vi "Session_Parser.vi"(8 "Error In":errorcluster, 11 "Consumer Data In":T2={"Queue_Consumer"=refnum, "Selected Consumer"=enum."Random", "Session Data"={"Tx-Data"=[], "Rx-Data"=[], "MIDI-Message log"=[{"Message Name"="", "Meta value"=0, "Datastring"="", "Datatype"=enum."No Data"}]}, "Timout-Time[ms]"=0, "To_GUI-Consumer"=refnum, "CPU(ms)"=0, "Console log"="", "MIDI Parse Data"={"MIDI-Bytes In"=[145, 60, 100], "MIDI Tag"=[], "MIDI Parsed Data"=[], "Iteration"=0, "Error?"=[], "Running States"=[], "Running Statusbyte"=0, "Running StatusString"="", "Third Byte Flag"=FALSE, "Current Byte"=0, "Sysex"="", "Expect Databyte"=FALSE}, "Session Inspection Data"={"Diff"=[], "Tx Byte"=[], "Rx Byte"=[], "Send Log"=[], "Parsed Data"={"Tx MIDI Tag"=[], "Tx MIDI Parsed Data"=[], "Tx Error"=[], "Tx Running States"=[], "Rx MIDI Tag"=[], "Rx MIDI Parsed Data"=[], "Rx Error"=[], "Rx Running States"=[], "Diff"=[]}}} {"MIDI Parse Data"."Current Byte" format="%.0x"; "MIDI Parse Data"."Running Statusbyte" format="%.0x"; "MIDI Parse Data"."MIDI-Bytes In" format="%.0x"}) -> (0 "Error Out":errorcluster, 3 "Consumer Data Out":T2={"Queue_Consumer"=refnum, "Selected Consumer"=enum."Random", "Session Data"={"Tx-Data"=[], "Rx-Data"=[], "MIDI-Message log"=[{"Message Name"="", "Meta value"=0, "Datastring"="", "Datatype"=enum."No Data"}]}, "Timout-Time[ms]"=0, "To_GUI-Consumer"=refnum, "CPU(ms)"=0, "Console log"="", "MIDI Parse Data"={"MIDI-Bytes In"=[145, 60, 100], "MIDI Tag"=[], "MIDI Parsed Data"=[], "Iteration"=0, "Error?"=[], "Running States"=[], "Running Statusbyte"=0, "Running StatusString"="", "Third Byte Flag"=FALSE, "Current Byte"=0, "Sysex"="", "Expect Databyte"=FALSE}, "Session Inspection Data"={"Diff"=[], "Tx Byte"=[], "Rx Byte"=[], "Send Log"=[], "Parsed Data"={"Tx MIDI Tag"=[], "Tx MIDI Parsed Data"=[], "Tx Error"=[], "Tx Running States"=[], "Rx MIDI Tag"=[], "Rx MIDI Parsed Data"=[], "Rx Error"=[], "Rx Running States"=[], "Diff"=[]}}} {"MIDI Parse Data"."Current Byte" format="%.0x"; "MIDI Parse Data"."Running Statusbyte" format="%.0x"; "MIDI Parse Data"."MIDI-Bytes In" format="%.0x"})   [LabVIEW 2019]
doc: "Description of VI"
uses:
  Controls/Consumer_Data.ctl
  Common/Controls/Application_Message.ctl
  Common/Controls/Application_State.ctl
  Controls/Consumer_States.ctl
  Controls/Transfer_Data.ctl
  MIDI/Controls/MIDI-Message_Array.ctl
  MIDI/Controls/MIDI-Message_Cluster.ctl
  MIDI/Controls/Meta_Commands.ctl
  Controls/Parser-data.ctl
  Controls/Consumer_Result.ctl
  Controls/Parsed_Data.ctl
  <vilib>/Utility/error.llb/DialogType.ctl
panel:
  out "Control Tab":T1(tab)
  out "Error Message":string
  out "VI-filename":string
  out "VI Path":path
  out "Code Size":u32
  out "Revision Number":u32
  in  "Tool Bar:Visible":bool
  in  "Tabs Visible?":bool
  out "VI-Name":string
  # "Settings"
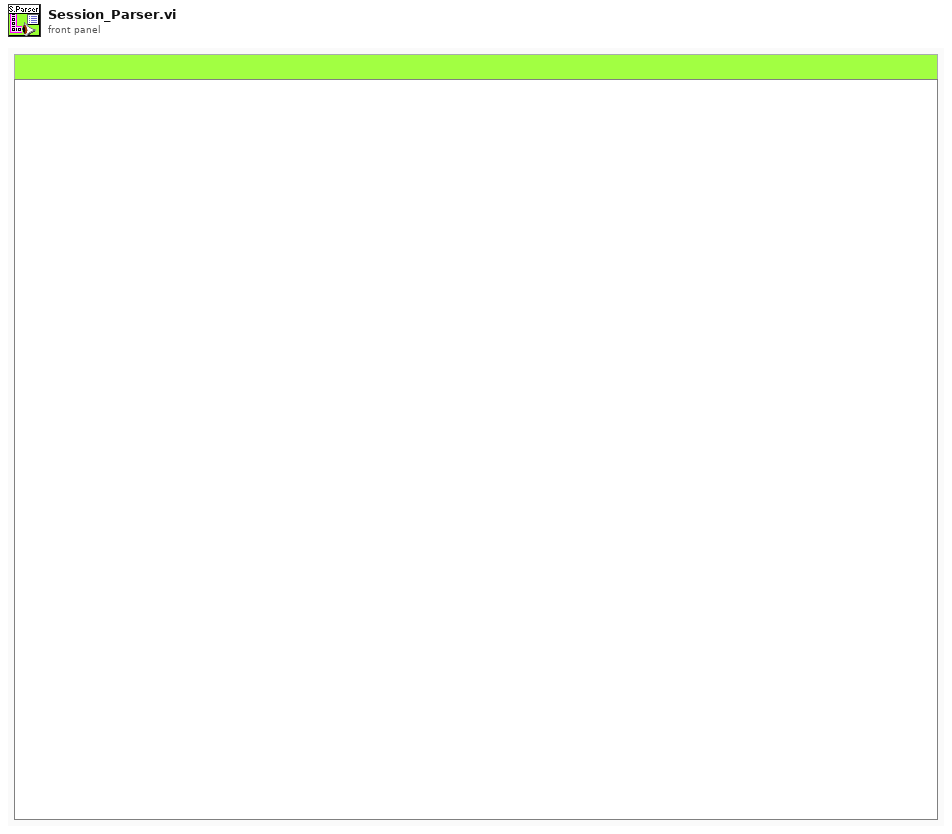
[diagram p1: front panel]
types:
  T1 = enum32{"GUI", "Console Log", "Controls & Indicators", "Data In", "Data Out", "Error IO", "VI"}
  T2 = typedef "Consumer_Data.ctl" = cluster{"Queue_Consumer":refnum<queue>, "Selected Consumer":T3, "Session Data":T4, "Timout-Time[ms]":i32, "To_GUI-Consumer":refnum<user-event>, "CPU(ms)":u32, "Console log":string, "MIDI Parse Data":T8, "Session Inspection Data":T9}
  T3 = typedef "Consumer_States.ctl" = enum16{"Random", "ECG", "Strech-Patch"}
  T4 = typedef "Transfer_Data.ctl" = cluster{"Tx-Data":i8[], "Rx-Data":i8[], "MIDI-Message log":T5}
  T5 = typedef "MIDI-Message_Array.ctl" = T6[]
  T6 = typedef "MIDI-Message_Cluster.ctl" = cluster{"Message Name":string, "Meta value":i32, "Datastring":string, "Datatype":T7}
  T7 = typedef "Meta_Commands.ctl" = enum16{"No Data", "Pause", "Loop", "Wait for Rx", "Delay", "Break", "MIDI"}
  T8 = typedef "Parser-data.ctl" = cluster{"MIDI-Bytes In":u8[], "MIDI Tag":string[], "MIDI Parsed Data":string[], "Iteration":i32, "Error?":bool[], "Running States":string[], "Running Statusbyte":u8, "Running StatusString":string, "Third Byte Flag":bool, "Current Byte":u8, "Sysex":string, "Expect Databyte":bool}
  T9 = typedef "Consumer_Result.ctl" = cluster{"Diff":bool[], "Tx Byte":string[], "Rx Byte":string[], "Send Log":string[], "Parsed Data":T10}
  T10 = typedef "Parsed_Data.ctl" = cluster{"Tx MIDI Tag":string[], "Tx MIDI Parsed Data":string[], "Tx Error":bool[], "Tx Running States":string[], "Rx MIDI Tag":string[], "Rx MIDI Parsed Data":string[], "Rx Error":bool[], "Rx Running States":string[], "Diff":bool[]}
  T11 = typedef "DialogType.ctl" = u16
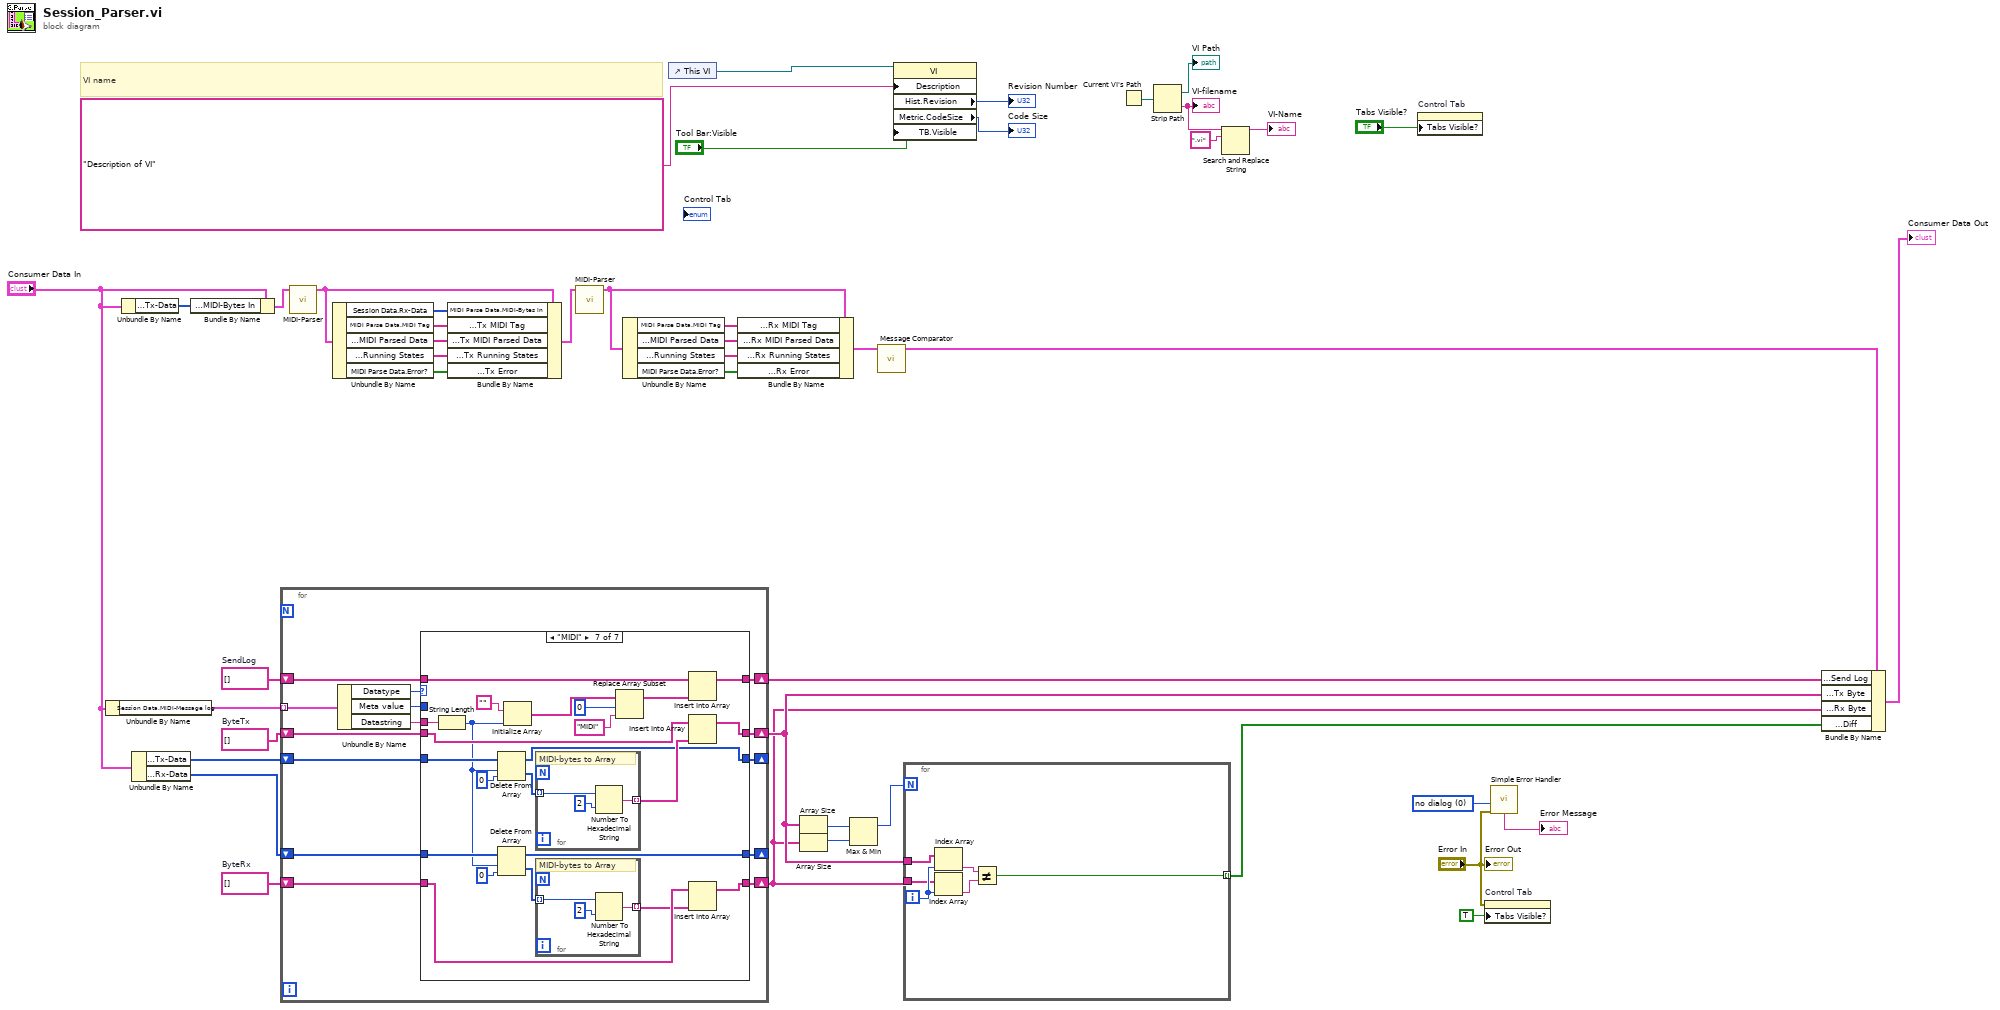
[diagram p0: block diagram]
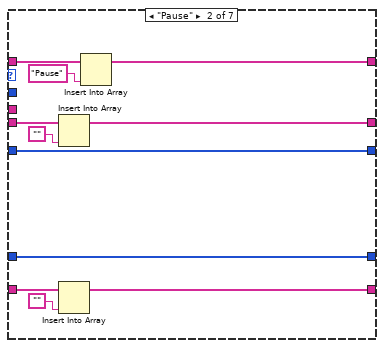
[diagram p3: hidden frame]
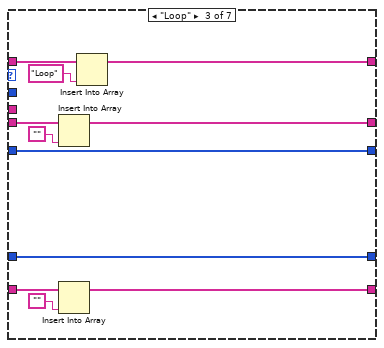
[diagram p4: hidden frame]
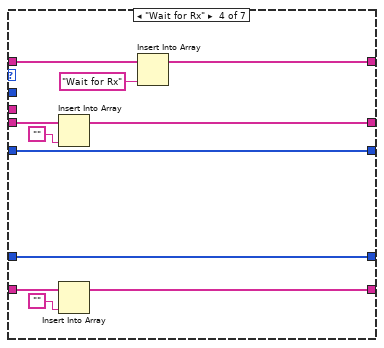
[diagram p5: hidden frame]
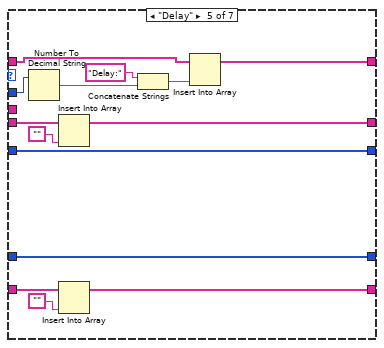
[diagram p6: hidden frame]
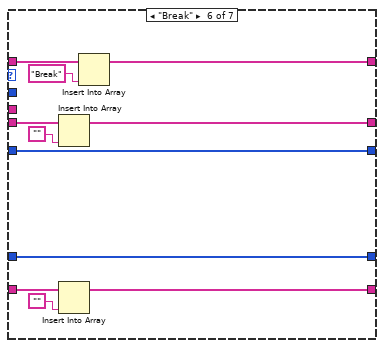
[diagram p7: hidden frame]
diagram:
  w26 = string[] []  # SendLog
  w27 = string[] []  # ByteRx
  w28 = string[] []  # ByteTx
  w37 = T11 0 items=["no dialog", "OK message", "continue or stop message", "OK message + warnings", "continue/stop + warnings"] ("type of dialog (OK msg:1)")
  # "VI name"
  n1 = Unbundle By Name("Consumer Data In") -> ("Session Data.MIDI-Message log"=w31:T5)
  n2 = Unbundle By Name("Consumer Data In") -> ("Session Data.Tx-Data"=w16:i8[])
  n3 = Unbundle By Name("Consumer Data In") -> ("Session Data.Tx-Data"=w30:i8[], "Session Data.Rx-Data"=w29:i8[])
  n4 = Bundle By Name(cluster="Consumer Data In", "MIDI Parse Data.MIDI-Bytes In"=w16) -> (w15:T2)
  n5 = for {
    tunnel: w31 -> [w60] mode=indexing
    shift-right: [w53] -> w20
    shift-left: w28 -> [w54]
    shift-right: [w51] -> w19
    shift-left: w27 -> [w52]
    shift-right: [w49] -> w25
    shift-left: w26 -> [w50]
    shift-right: [w48] -> _
    shift-left: w30 -> [w56]
    shift-right: [w47] -> _
    shift-left: w29 -> [w55]
    n6 = Unbundle By Name(w60) -> ("Datatype"=w59:T7, "Meta value"=w58:i32, "Datastring"=w57:string)
    n7 = case shown="\"MIDI\"" w59 {
      tunnel: w58 -> [_ _ _ _ w111 _ _]
      tunnel: w57 -> [_ _ _ _ _ _ w146]
      tunnel: w56 -> [w62 w67 w78 w89 w100 w114 w145]
      tunnel: w55 -> [w61 w66 w77 w88 w99 w113 w144]
      tunnel: w54 -> [w65 w76 w86 w97 w108 w122 w140]
      tunnel: [w65 w75 w85 w96 w107 w121 w139] -> w53
      tunnel: w52 -> [w64 w74 w83 w94 w105 w119 w138]
      tunnel: [w64 w73 w82 w93 w104 w118 w137] -> w51
      tunnel: w50 -> [w63 w70 w81 w91 w102 w117 w131]
      tunnel: [w63 w69 w80 w92 w103 w116 w130] -> w49
      tunnel: [w62 w67 w78 w89 w100 w114 w127] -> w48
      tunnel: [w61 w66 w77 w88 w99 w113 w126] -> w47
      frame "No Data", Default {
      }
      frame "Pause" {
        n8 = Insert Into Array(array=w76, new element="") -> (w75:string[])  [unwired: 1 in]
        n9 = Insert Into Array(array=w74, new element="") -> (w73:string[])  [unwired: 1 in]
        n10 = Insert Into Array(array=w70, new element="Pause") -> (w69:string[])  [unwired: 1 in]
      }
      frame "Loop" {
        n11 = Insert Into Array(array=w86, new element="") -> (w85:string[])  [unwired: 1 in]
        n12 = Insert Into Array(array=w83, new element="") -> (w82:string[])  [unwired: 1 in]
        n13 = Insert Into Array(array=w81, new element="Loop") -> (w80:string[])  [unwired: 1 in]
      }
      frame "Wait for Rx" {
        n14 = Insert Into Array(array=w97, new element="") -> (w96:string[])  [unwired: 1 in]
        n15 = Insert Into Array(array=w94, new element="") -> (w93:string[])  [unwired: 1 in]
        n16 = Insert Into Array(array=w91, new element="Wait for Rx") -> (w92:string[])  [unwired: 1 in]
      }
      frame "Delay" {
        n17 = Number To Decimal String(number=w111) -> (decimal integer string=w110:string)  [unwired: 1 in]
        n18 = Insert Into Array(array=w108, new element="") -> (w107:string[])  [unwired: 1 in]
        n19 = Insert Into Array(array=w105, new element="") -> (w104:string[])  [unwired: 1 in]
        n20 = Concatenate Strings("Delay:", w110) -> (w101:string)
        n21 = Insert Into Array(array=w102, new element=w101) -> (w103:string[])  [unwired: 1 in]
      }
      frame "Break" {
        n22 = Insert Into Array(array=w122, new element="") -> (w121:string[])  [unwired: 1 in]
        n23 = Insert Into Array(array=w119, new element="") -> (w118:string[])  [unwired: 1 in]
        n24 = Insert Into Array(array=w117, new element="Break") -> (w116:string[])  [unwired: 1 in]
      }
      frame "MIDI" {
        n25 = String Length(string=w146) -> (length=w128:i32)
        n26 = Delete From Array(array=w145, length=w128, index=0) -> (deleted portion=w141:i8[], array with subset deleted=w127:i8[])
        n27 = Delete From Array(array=w144, length=w128, index=0) -> (deleted portion=w124:i8[], array with subset deleted=w126:i8[])
        n28 = Initialize Array("", w128) -> (w135:string[])
        n29 = for {
          tunnel: w141 -> [w150] mode=indexing
          tunnel: [w151] -> w129 mode=indexing
          # "MIDI-bytes to Array"
          n30 = Number To Hexadecimal String(1:i16 2 ("width (-)"), 2:w150) -> (0:w151:string)
        }
        n31 = for {
          tunnel: w124 -> [w147] mode=indexing
          tunnel: [w148] -> w125 mode=indexing
          # "MIDI-bytes to Array"
          n32 = Number To Hexadecimal String(1:i16 2 ("width (-)"), 2:w147) -> (0:w148:string)
        }
        n33 = Replace Array Subset(array=w135, new element="MIDI", index=0) -> (w132:string[])
        n34 = Insert Into Array(array=w131, new element=w132) -> (w130:string[])  [unwired: 1 in]
        n35 = Insert Into Array(array=w140, new element=w129) -> (w139:string[])  [unwired: 1 in]
        n36 = Insert Into Array(array=w138, new element=w125) -> (w137:string[])  [unwired: 1 in]
      }
    }
  }
  n37 = call "MIDI-Parser.vi"("Consumer Data In"=w15) -> ("Consumer Data Out"=w13:T2)  [unwired: 9 in, 1 out]
  n38 = Unbundle By Name(w13) -> ("Session Data.Rx-Data"=w14:i8[], "MIDI Parse Data.MIDI Tag"=w12:string[], "MIDI Parse Data.MIDI Parsed Data"=w11:string[], "MIDI Parse Data.Running States"=w10:string[], "MIDI Parse Data.Error?"=w9:bool[])
  n39 = Bundle By Name(cluster=w13, "MIDI Parse Data.MIDI-Bytes In"=w14, "Session Inspection Data.Parsed Data.Tx MIDI Tag"=w12, "Session Inspection Data.Parsed Data.Tx MIDI Parsed Data"=w11, "Session Inspection Data.Parsed Data.Tx Running States"=w10, "Session Inspection Data.Parsed Data.Tx Error"=w9) -> (w8:T2)
  n40 = call "MIDI-Parser.vi"("Consumer Data In"=w8) -> ("Consumer Data Out"=w7:T2)  [unwired: 9 in, 1 out]
  n41 = Unbundle By Name(w7) -> ("MIDI Parse Data.MIDI Tag"=w6:string[], "MIDI Parse Data.MIDI Parsed Data"=w5:string[], "MIDI Parse Data.Running States"=w4:string[], "MIDI Parse Data.Error?"=w3:bool[])
  n42 = control-ref of="This VI"() -> (w43:refnum<vi>)
  n43 = Bundle By Name(cluster=w7, "Session Inspection Data.Parsed Data.Rx MIDI Tag"=w6, "Session Inspection Data.Parsed Data.Rx MIDI Parsed Data"=w5, "Session Inspection Data.Parsed Data.Rx Running States"=w4, "Session Inspection Data.Parsed Data.Rx Error"=w3) -> (w1:T2)
  n44 = Array Size(array=w20) -> (size(s)=w23:i32)
  n45 = Array Size(array=w19) -> (size(s)=w22:i32)
  n46 = Max & Min(x=w23, y=w22) -> (max(x,y)=w21:i32)  [unwired: 1 out]
  n47 = call "Message Comparator.vi"("Consumer Data Out in"=w1) -> ("Consumer Data Out out"=w2:T2)  [unwired: 10 in]
  n48 = property class="VI"(reference=w43, "Description"="Description of VI", "TB.Visible"="Tool Bar:Visible") -> ("Hist.Revision"=→"Revision Number":u32, "Metric.CodeSize"=→"Code Size":u32)  [unwired: 1 in, 2 out]
  n49 = for {
    N: w21 -> [_]
    tunnel: w20 -> [w157]
    tunnel: w19 -> [w156]
    tunnel: [w153] -> w18 mode=indexing
    i -> [w158]
    n50 = Index Array(array=w157, index=w158) -> (element=w155:string)
    n51 = Index Array(array=w156, index=w158) -> (element=w154:string)
    n52 = Not Equal?(x=w155, y=w154) -> (x != y?=w153:bool)
  }
  n53 = Current VI's Path() -> (path=w46:path)
  n54 = Strip Path(path=w46) -> (stripped path=→"VI Path":path, name=w40:string)
  "VI-filename" <- w40
  n55 = Search and Replace String(input string=w40, search string=".vi") -> (result string=→"VI-Name":string)  [unwired: 6 in, 3 out]
  n56 = property on="Control Tab" class="TabCtl (strict)"("Tabs Visible?"="Tabs Visible?") -> ()  [unwired: 2 in, 2 out]
  n57 = property on="Control Tab" class="TabCtl (strict)"(error in="Error In", "Tabs Visible?"=TRUE) -> ()  [unwired: 1 in, 2 out]
  n58 = call <vilib>:"Simple Error Handler.vi"("type of dialog (OK msg:1)"=w37, "error in (no error)"="Error In") -> ("message"=→"Error Message":string)  [unwired: 3 in, 4 out]
  n59 = Bundle By Name(cluster=w2, "Session Inspection Data.Send Log"=w25, "Session Inspection Data.Tx Byte"=w20, "Session Inspection Data.Rx Byte"=w19, "Session Inspection Data.Diff"=w18) -> (→"Consumer Data Out":T2)
  "Error Out" <- "Error In"
